vi "Blynk Virtual Write.vi"(8 "error in":errorcluster, 9 "value":string, 10 "pin":string, 11 "connection":refnum<k5>) -> (0 "error out":errorcluster, 3 "connection out":refnum<k5>)   [LabVIEW 2014]
uses:
  utilities/MsgType.ctl
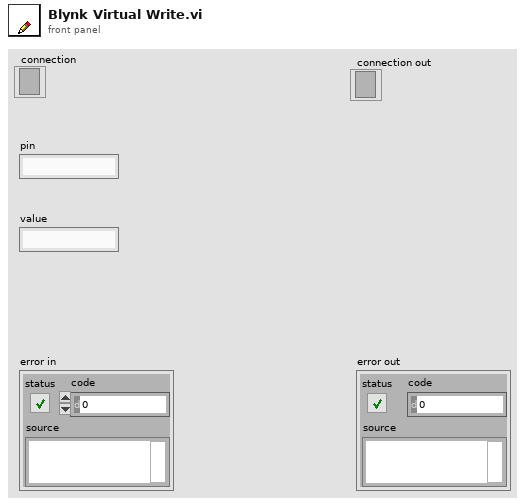
[diagram p1: front panel]
types:
  T1 = typedef "MsgType.ctl" = enum8{"RSP", "REGISTER", "LOGIN", "SAVE_PROF", "LOAD_PROF", "GET_TOKEN", "PING", "ACTIVATE", "DEACTIVATE", "REFRESH", "UNDEFINED0", "UNDEFINED1", "TWEET", "EMAIL", "NOTIFY", "BRIDGE", "UNDEFINED2", "UNDEFINED3", "UNDEFINED4", "UNDEFINED5", "HW"}
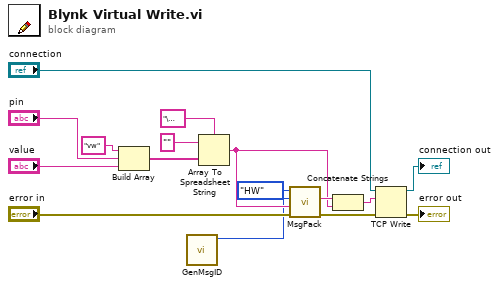
[diagram p0: block diagram]
diagram:
  n1 = Build Array("vw" ("format string"), "pin", "value") -> (w8:string[])
  n2 = call "GenMsgID.vi"() -> ("MsgID"=w1:u16)  [unwired: 10 in, 1 out]
  n3 = Array To Spreadsheet String(delimiter (Tab)="\u0000", array=w8, 3:"" ("format string")) -> (spreadsheet string=w13:string)
  n4 = call "MsgPack.vi"("error in"="error in", "msg"=w13, "msg_id"=w1, "msg_type"=MsgType."HW") -> ("error out"=w11:errorcluster, "msg_data"=w14:string)  [unwired: 6 in]
  n5 = Concatenate Strings(w14, w13) -> (w12:string)
  n6 = TCP Write(connection ID="connection", data in=w12, error in (no error)=w11) -> (connection ID out=→"connection out":refnum<k5>, error out=→"error out":errorcluster)  [unwired: 1 in, 1 out]
